vi "Virtual Camera Stop Live Mode.vi"(8 "error in (no error)":errorcluster, 11 "Virtual Camera in":refnum<class "Virtual Camera.lvclass">) -> (0 "error out":errorcluster, 3 "Virtual Camera out":refnum<class "Virtual Camera.lvclass">)   [LabVIEW 2015, in "Virtual Camera.lvlib" / "Virtual Camera.lvclass"]
uses:
  Virtual Camera.lvclass
  Orca-Flash 4.0 V2 Messages/Flash Stop Live Mode Msg/Flash Stop Live Mode Msg.lvclass
  <vilib>/ActorFramework/Stop Msg/Stop Msg.lvclass
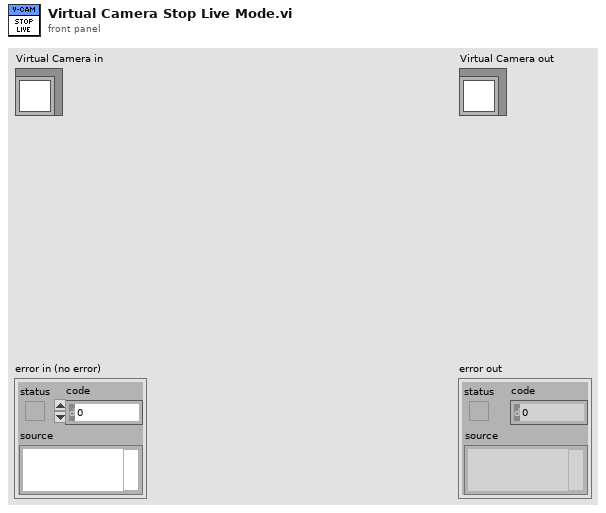
[diagram p1: front panel]
types:
  T1 = typedef "Semaphore RefNum" = refnum<k1>
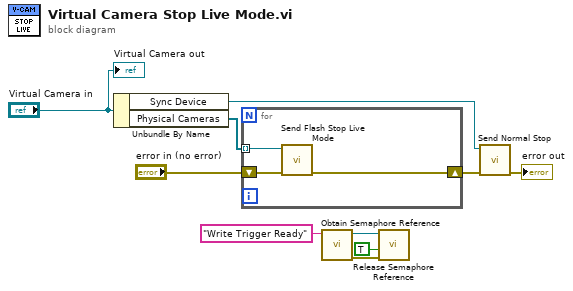
[diagram p0: block diagram]
diagram:
  n1 = Unbundle By Name("Virtual Camera in") -> ("Sync Device"=w7:refnum<class "Message Enqueuer.lvclass">, "Physical Cameras"=w10:refnum<class "Message Enqueuer.lvclass">[])
  n2 = for {
    tunnel: w10 -> [w12] mode=indexing
    shift-right: [w11] -> w6
    shift-left: "error in (no error)" -> [w13]
    n3 = call "Send Flash Stop Live Mode.vi"("error in (no error)"=w13, "Message Enqueuer"=w12) -> ("error out"=w11:errorcluster)  [unwired: 8 in, 1 out]
  }
  n4 = call <vilib>:"Obtain Semaphore Reference.vi"("name (unnamed)"="Write Trigger Ready") -> ("error out"=w3:errorcluster, "semaphore"=w2:T1)  [unwired: 4 in, 1 out]
  n5 = call <vilib>:"Release Semaphore Reference.vi"("error in (no error)"=w3, "force destroy? (F)"=TRUE, "semaphore"=w2) -> ()  [unwired: 7 in, 2 out]
  n6 = call <vilib>:"Send Normal Stop.vi"("error in (no error)"=w6, "Message Enqueuer"=w7) -> ("error out"=→"error out":errorcluster)  [unwired: 9 in]
  "Virtual Camera out" <- "Virtual Camera in"
